vi "Shooter_Fire_1_20.vi"(8 "CamPos":dbl, 9 "PotPos In":dbl, 10 "FireButton":bool, 11 "IsReady":bool) -> (0 "CamPow":dbl, 1 "CamPosOut":dbl, 3 "PotPosOut":dbl)   [LabVIEW 2013]
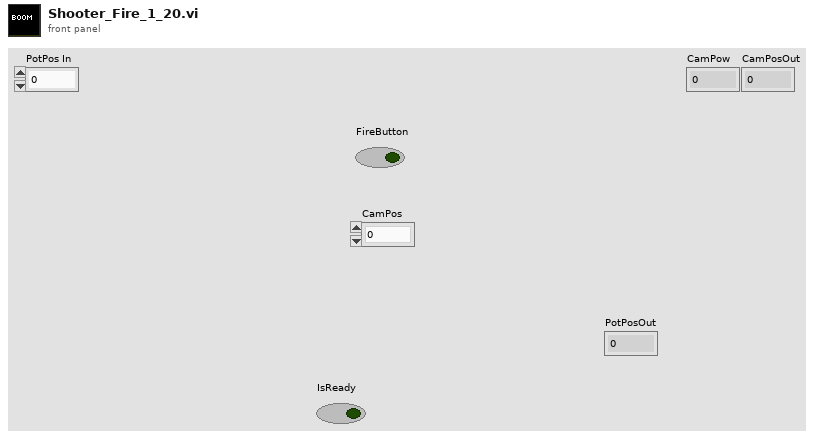
[diagram p1: front panel]
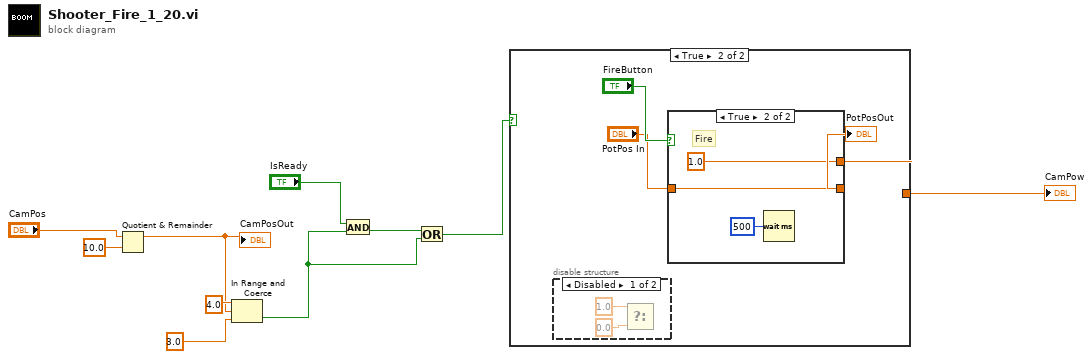
[diagram p0: block diagram]
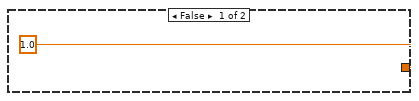
[diagram p2: hidden frame]
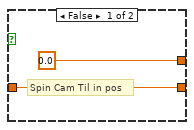
[diagram p4: hidden frame]
diagram:
  n1 = Quotient & Remainder(x="CamPos", y=10.0) -> (x-y*floor(x/y)=w4:dbl)  [unwired: 1 out]
  "CamPosOut" <- w4
  n2 = In Range and Coerce(upper limit=4.0 ("x"), x=w4, lower limit=3.0 ("y")) -> (In Range?=w2:bool)  [unwired: 1 out]
  n3 = And(x="IsReady", y=w2) -> (x .and. y?=w7:bool)
  n4 = Or(x=w7, y=w2) -> (x .or. y?=w6:bool)
  n5 = case shown="True" w6 {
    tunnel: [1.0 ("CamPower") w12] -> w1
    frame False {
    }
    frame True {
      n6 = disable-structure shown="Disabled" {
        frame Disabled {
          n7 = Select(t=1.0, f=0.0) -> ()  [unwired: 1 in, 1 out]
        }
        frame Enabled {
        }
      }
      n8 = case shown="True" "FireButton" {
        tunnel: [w19 w20] -> w14
        tunnel: "PotPos In" -> [w19 w20]
        tunnel: [0.0 ("CamPos") 1.0 ("CamPower")] -> w12
        frame False {
          # "Spin Cam Til in pos"
        }
        frame True {
          # "Fire"
          n9 = Wait (ms)(milliseconds to wait=u32 500) -> ()  [unwired: 1 out]
        }
      }
      "PotPosOut" <- w14
    }
  }
  "CamPow" <- w1
